vi "glb_DataLog MCVD.vi"() -> ()   [LabVIEW 2012]
doc: "Data logging constants set via \"make current value default\". Do not change these values once a system has been deployed. This will affect the tag logging storage format and naming scheme, thus rendering the system incompatible with data logged using the previous configuration."
uses:
  typedefs/clusters/t_DataLog Tag Config.ctl
  typedefs/t_DataLog Temporal Types.ctl
  typedefs/t_DataLog Value Types.ctl
  typedefs/t_DataLog Numerical Format.ctl
  typedefs/t_DataLog Logging Algorithms.ctl
panel:
  in  "subset file":string="subsets.lua"
  in  "warning logsize limit":dbl=137438953472.0
  in  "NaN string":string="UNDEFINED"
  in  "default config":T1={"name"="", "unit"="", "temporal"=enum."sample", "value"=enum."number", "index"=0, "capacity"=0, "is meta?"=FALSE, "mincapacity"=0, "deadband"=0.0, "limit delay"=0.0, "format"=enum."fractional", "precision"=6, "undefine"=FALSE, "update"=FALSE, "update period"=0, "expression"="", "description"="", "logging algorithm"=enum."nothing", "logging parameters"=[]} {"logging parameters" format="%.2e"; "precision" items=["0", "1", "2", "3", "4", "5", "6", "7", "8", "9", "10", "11", "12", "13", "14", "15", "16", "17"]; "limit delay" format="%.2e"; "deadband" format="%.2e"}
  in  "bytes per point":i32=16
  in  "bytes per double":i32=8
  in  "warning strings file size":dbl=2000000000.0
  in  "max strings file size":dbl=2147000000.0
  in  "strings file name":string="strings.dat"
  in  "tag config file name":string="config.lua"
  in  "recovery file":string="recovery.dat"
  in  "hash file":string="tag_hash.dat"
  in  "points per chunk":dbl=16384.0
  in  "chunks per file":dbl=4096.0
  in  "points file format":string="points%04d.dat"
  in  "index file name":string="index.dat"
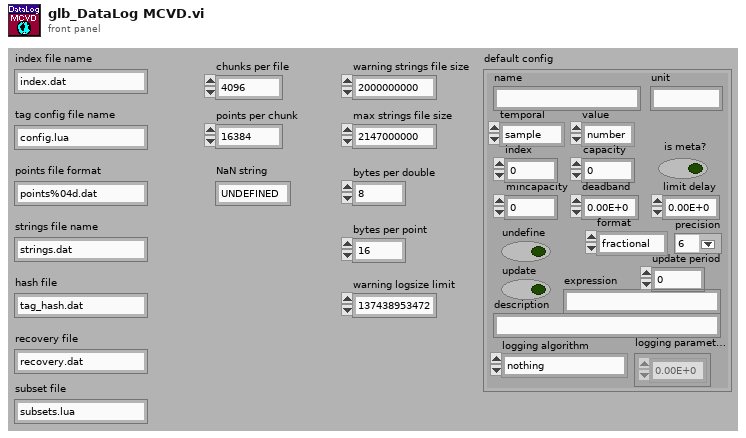
[diagram p1: front panel]
types:
  T1 = typedef "t_DataLog Tag Config.ctl" = cluster{"name":string, "unit":string, "temporal":T2, "value":T3, "index":i32, "capacity":i32, "is meta?":bool, "mincapacity":i32, "deadband":dbl, "limit delay":dbl, "format":T4, "precision":u8, "undefine":bool, "update":bool, "update period":u16, "expression":string, "description":string, "logging algorithm":T5, "logging parameters":dbl[]}
  T2 = typedef "t_DataLog Temporal Types.ctl" = enum16{"set&hold", "sample", "event"}
  T3 = typedef "t_DataLog Value Types.ctl" = enum16{"number", "string"}
  T4 = typedef "t_DataLog Numerical Format.ctl" = enum8{"fractional", "exponential", "engineering"}
  T5 = typedef "t_DataLog Logging Algorithms.ctl" = enum16{"nothing", "changes", "everything", "every Nth", "time threshold", "value threshold + prior", "t or v threshold", "t or v threshold + prior"}
diagram:
